vi "is Empty.vi"(4 "JSON":string) -> (1 "Empty":bool)   [LabVIEW 2021, in "json.facade.lvlib"]
doc: "Returns TRUE if the input text starts with any of these JSON types that are \"empty\":\n1) null\n2) NaN\n3) \"\" (an empty JSON string)\n4) A JSON Object containing no items\n5) An empty JSON Array \n6) no JSON at all (empty string or only whitespace)\n\nReturns False if the input starts with non-empty JSON.\n\nThis function will return FALSE if it detects invalid JSON, but as it only inspects the lead characters, it cannot be relied on to validate the input as proper JSON."
uses:
  json.facade.lvlib
  jsontext/JSONtext.lvlib
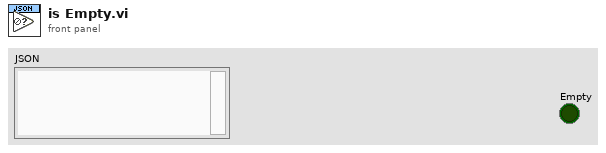
[diagram p1: front panel]
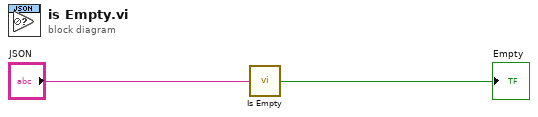
[diagram p0: block diagram]
diagram:
  n1 = call "Is Empty.vi"("JSON"="JSON") -> ("Empty"=→"Empty":bool)  [unwired: 4 in]
